vi "DecodeHeader.vi"(7 "WPILOG_Version":i16=1, 11 "wpilog (bytes)":u8[](array[numeric])) -> (1 "extra header string":string, 3 "rest of the log":u8[](array[numeric]))   [LabVIEW 2023]
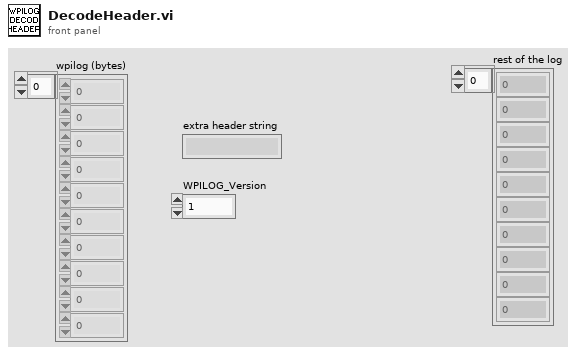
[diagram p1: front panel]
types:
  T1 = enum16{"big-endian, network order", "native, host order", "little-endian"}
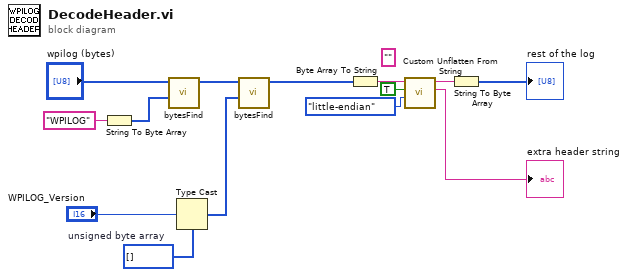
[diagram p0: block diagram]
diagram:
  (unwired) ""
  w13 = u8[] []  # unsigned byte array
  n1 = String To Byte Array(string="WPILOG") -> (unsigned byte array=w10:u8[])
  n2 = call "bytesFind.vi"("find bytes"=w10, "log"="wpilog (bytes)") -> ("rest of the log"=w9:u8[])  [unwired: 7 in, 2 out]
  n3 = Type Cast(type=w13, x="WPILOG_Version") -> (*(type *) &x=w8:u8[])
  n4 = call "bytesFind.vi"("find bytes"=w8, "log"=w9) -> ("rest of the log"=w7:u8[])  [unwired: 7 in, 2 out]
  n5 = Byte Array To String(unsigned byte array=w7) -> (string=w5:string)
  n6 = call "Custom Unflatten From String.vi"("byte order (0:big-endian, network order)"=T1."little-endian", "data includes array or string size? (T)"=TRUE, "binary string"=w5) -> ("value"=→"extra header string":string, "rest of the binary string"=w4:string)  [unwired: 7 in]
  n7 = String To Byte Array(string=w4) -> (unsigned byte array=→"rest of the log":u8[])
